vi "p2.vi"() -> ()   [LabVIEW 2023, in "d8.lvlib"]
uses:
  d8.lvlib
  <vilib>/Utility/error.llb/Trim Whitespace One-Sided.vi
  AOC/AOC.lvlib
panel:
  in  "Input":string="LRRLRRRLRRRLLRRLRRLRLRLRRLLRRLRRLRRRLLLRRRLRRRLRRRLLRRRLRRLLRRLRRLRLRRRLRRLRLRRLRRRLLRRLLRLRRRLLRRLRRLLLRLRRRLRLRLRLLRRRLRLLRRRLRLRRRLRRRLLRRLRRRLLRRLRLLRLRRLLLRRLRRLLLRLLRLRRRLRLRLRRRLRRLLRRRLRLRLRRLRRRLRLRRLRRLRRRLRRRLRRRLRRRLRRLLRRLRLLRRLLRRRLRLLRLRLRRLRRLRLRLRRRLRLRLRRLRLRRLRRRR\n\nFPF = (PTN, MPT)\nDGM = (KXM, PRM)\nFKB = (JLC, MBX)\nXCJ = (DCJ, TSH)\nJVH = (VCH, SMV)\nBXL = (HLB, NVF)\nGVD = (FSQ, MFD)\nCDJ = (SMM, HHS)\nBGM = (FHB, LKH)\nFBP = (HHS, SMM)\nLTK = (TCV, GQX)\nLDM = (MRM, JKJ)\nRDK = (KBL, GHP)\nBJB = (XBN, BXG)\nKST = (BGX, VFS)\nVKM = (MFR, CJP)\nCSG = (GGJ, JHH)\nJFS = (QCG, XFR)\nMDV = (FPQ, NRX)\nQHF = (PJP, QHX)\nDHM = (LJC, PDS)\nMMV = (CHS, FXX)\nCQP = (LFN, GSD)\nRDT = (NVG, NVG)\nXFN = (HFM, LTK)\nMFD = (RKJ, XGN)\nDTD = (JBV, JBV)\nKJG = (PCC, PPR)\nGLH = (JRN, BLK)\nKBV = (MCQ, MCS)\nLQF = (KDR, GFC)\nGGB = (JGL, RRM)\nBQX = (QKQ, NSG)\nSVS = (SQL, FXL)\nGMC = (BHG, GPC)\nKPZ = (HLV, RVH)\nRQB = (TDV, XPN)\nGVR = (SXD, QRB)\nMNX = (DLT, CMJ)\nQDM = (TKN, VDH)\nCCB = (KPR, QCK)\nBVF = (QJX, FKK)\nTJB = (HKV, BCP)\nBHC = (SSN, HHH)\nNTN = (RPT, PVF)\nNDP = (BJQ, MGH)\nPJP = (NTN, FSR)\nBLL = (MTQ, SNQ)\nRNP = (RTD, PGM)\nPVF = (BMP, LPM)\nQFL = (NNS, GLR)\nVRG = (GGV, DMG)\nXRX = (TTR, LXS)\nMBH = (RHX, GKF)\nCXD = (LFN, GSD)\nFFK = (LDG, VHS)\nNHM = (BLM, XQD)\nTNB = (KSS, FSB)\nVLX = (KCF, VXL)\nDDF = (TNK, FBS)\nGQR = (BGM, MGR)\nBPQ = (FHD, MJT)\nKPR = (SDL, NMQ)\nCNL = (QFP, XPV)\nHVA = (BRQ, XPL)\nPHF = (LHF, HVR)\nTNZ = (XCM, BFL)\nNDJ = (GCQ, RTL)\nHCT = (PQT, VVB)\nJNH = (GVV, JMC)\nCNV = (SDP, NQR)\nGGV = (RHT, SLG)\nPRX = (FSD, KST)\nBLM = (KKQ, CSG)\nJRN = (GGK, GBF)\nDJK = (GQJ, JKB)\nRVH = (FXJ, JVN)\nRXF = (CHG, GDT)\nMBX = (KJM, XFN)\nHLV = (JVN, FXJ)\nXDG = (HJM, KCT)\nLPM = (RCG, RHG)\nGLP = (XDM, XNC)\nHQP = (JXQ, XPT)\nCXF = (SCV, PHF)\nQJT = (FJN, GHV)\nMPL = (HSQ, FKN)\nSDP = (LCQ, GRV)\nCDQ = (JLV, LLD)\nHHA = (BFL, XCM)\nGPS = (VLX, CPL)\nBXZ = (KSN, VKP)\nPGM = (LJV, CDQ)\nPKG = (VQF, FXC)\nXPL = (LBN, DMV)\nBJJ = (TVV, MNX)\nHLB = (SNN, HNH)\nCDV = (TNB, FSN)\nFXC = (CLF, HSC)\nJFM = (LSR, CNL)\nCMV = (DHQ, DJR)\nLDN = (BCQ, JMS)\nXNC = (JLS, KXS)\nSNN = (NGM, MFJ)\nCND = (RDL, GJJ)\nSKT = (FCM, MRC)\nQRB = (BCG, HRR)\nXNK = (LJC, PDS)\nDGK = (KBF, SRB)\nLNL = (FSD, KST)\nPCM = (PDL, JFS)\nBSV = (LSR, CNL)\nSMX = (TKL, QPF)\nXMS = (MDB, PKP)\nXPT = (LDM, PKV)\nRLB = (XFT, PKM)\nVVV = (NRX, FPQ)\nMGB = (LNN, NKR)\nSFJ = (LFT, QDM)\nMFX = (GLP, RPN)\nDLX = (SQQ, NHM)\nXQC = (HQJ, NPC)\nGHF = (VNG, TGQ)\nLRX = (GDT, CHG)\nSHV = (SRM, DVJ)\nTQS = (PRD, HGV)\nSQK = (QNB, PSJ)\nCHS = (MXK, GCR)\nVDH = (FMX, XMR)\nDGN = (LGT, PNQ)\nRMM = (CFK, RQD)\nRQK = (FSN, TNB)\nSLH = (BDS, BBP)\nHVR = (NTS, NQG)\nPSJ = (JFK, XXM)\nGBD = (VMR, KJG)\nFRH = (MNX, TVV)\nTHH = (GHF, MNF)\nXTP = (VPC, BQQ)\nVMR = (PCC, PPR)\nPPQ = (GJJ, RDL)\nVHK = (TXT, DDN)\nJCG = (CCD, BXL)\nLCQ = (MPF, NDP)\nKCR = (PFH, DJK)\nLHL = (LGL, KCR)\nJMC = (RBG, CGH)\nJPM = (XMS, CVR)\nCLF = (HDT, DHR)\nFSQ = (XGN, RKJ)\nDVJ = (VHD, XNM)\nKCT = (SKT, QLK)\nXFD = (HXR, JVH)\nBVA = (GPT, RSD)\nMGR = (FHB, LKH)\nPXV = (MJJ, VBK)\nFNG = (TQS, HHM)\nGFD = (XRG, JCS)\nSST = (PHP, JGC)\nKJV = (DMG, GGV)\nPQM = (TTX, RMM)\nXRT = (KBL, GHP)\nJLV = (NKV, BLL)\nFKS = (CBR, RLJ)\nHMD = (JNH, GXG)\nFRL = (KQX, DDB)\nTRP = (LXT, HMC)\nTNK = (FRN, FRN)\nKDR = (PRX, LNL)\nXTS = (NDJ, HFB)\nHVM = (FMG, FHN)\nCHH = (TMD, MNM)\nHHM = (PRD, HGV)\nPJC = (FCC, VJD)\nTSH = (RPR, CVJ)\nGGJ = (NFK, NXD)\nDMG = (RHT, SLG)\nQPT = (QFL, PFN)\nDDN = (RHP, NSS)\nXHJ = (BPQ, CSM)\nNNM = (KHG, SRF)\nLFL = (TMN, JCG)\nNKV = (SNQ, MTQ)\nTMH = (LGT, PNQ)\nCCD = (HLB, NVF)\nGSD = (MRB, TFS)\nRHG = (VXH, MXS)\nLFT = (TKN, VDH)\nBJV = (DST, PTK)\nCGD = (PKG, ZZZ)\nVNG = (BJV, HDX)\nHJS = (GPC, BHG)\nFRN = (VKP, KSN)\nMRC = (JKK, CMV)\nBQQ = (NBF, PJC)\nKSN = (FNJ, GVR)\nQNB = (XXM, JFK)\nRSC = (JCB, JCB)\nGCQ = (XGH, FKB)\nSHS = (JBV, DDF)\nLLR = (XHJ, PGB)\nRSA = (RVH, HLV)\nDMX = (GSH, SST)\nHRD = (HLK, DJG)\nLHF = (NTS, NQG)\nJMS = (FKS, HPB)\nSRB = (SRG, GSF)\nLHN = (HLK, DJG)\nDTM = (RXM, VHK)\nPNP = (SNC, LPF)\nMPF = (BJQ, BJQ)\nSCV = (LHF, HVR)\nBTV = (GLH, PNN)\nNJG = (RXK, NXB)\nNGM = (THG, TXQ)\nFXL = (XRX, MBV)\nNHJ = (DSX, NNM)\nRBG = (DGK, LFQ)\nHGV = (HTS, RNP)\nLDF = (KRB, NXC)\nPMR = (GNH, CHQ)\nDVM = (MNM, TMD)\nFBS = (FRN, BXZ)\nBMM = (XSK, DDK)\nGGK = (MXH, JNG)\nNXB = (LHN, HRD)\nPNN = (JRN, BLK)\nPSV = (LLR, KXX)\nKGK = (TJP, QMM)\nCVG = (VLX, CPL)\nQNF = (XPB, PCM)\nHTS = (PGM, RTD)\nFJN = (DTD, SHS)\nJXB = (CLX, KPZ)\nDLT = (JGH, SFD)\nSFV = (HJM, KCT)\nGSF = (DLX, CHL)\nTKN = (XMR, FMX)\nLJB = (QJT, FVJ)\nQFP = (NXL, DGP)\nPKV = (JKJ, MRM)\nRHX = (RDK, XRT)\nKDP = (FKN, HSQ)\nRLJ = (BGF, JRP)\nVQR = (FDK, RLB)\nXNX = (HGQ, HGQ)\nDSX = (KHG, SRF)\nPDS = (VQK, KNJ)\nGKX = (TKL, QPF)\nCHQ = (XSM, HMD)\nKXX = (XHJ, PGB)\nMDB = (VVV, MDV)\nBCG = (XJX, SQK)\nKJM = (LTK, HFM)\nHRR = (SQK, XJX)\nGXD = (JFM, BSV)\nSCR = (JDN, QRS)\nGMK = (FPF, CTM)\nKXM = (PDJ, MFX)\nDKQ = (GCL, QFN)\nDJR = (FGV, PSV)\nGQX = (DFL, LQF)\nPTK = (TRS, TMC)\nBLK = (GGK, GBF)\nRSD = (XDG, SFV)\nSVT = (PXV, XCL)\nXFT = (BJJ, FRH)\nLSR = (XPV, QFP)\nBCP = (NMB, NXM)\nKGP = (RDT, FNB)\nDHF = (PNN, GLH)\nJHH = (NXD, NFK)\nDGP = (GKX, SMX)\nKSK = (DKP, RXT)\nKRM = (PQM, DCK)\nXJX = (QNB, PSJ)\nJKK = (DJR, DHQ)\nCFK = (DGN, TMH)\nPSS = (HNP, STL)\nMFR = (PMR, RJS)\nJNG = (TQQ, HXB)\nMDG = (VCC, HTF)\nVCC = (DGM, MKH)\nTQQ = (FCQ, SCR)\nDMK = (GXD, GFF)\nGHV = (DTD, SHS)\nHLP = (NNH, TQN)\nBGK = (QHJ, BQX)\nVKN = (DPT, FNG)\nSTL = (DPP, NMX)\nQFS = (MGR, BGM)\nHSC = (DHR, HDT)\nFPQ = (NSL, RQN)\nQMM = (CDJ, FBP)\nPDL = (XFR, QCG)\nPDJ = (GLP, RPN)\nFSD = (VFS, BGX)\nMPT = (DKQ, RSQ)\nMHQ = (NTL, TKG)\nMPC = (NQJ, NQJ)\nDST = (TRS, TMC)\nKHD = (CLX, CLX)\nBNT = (MFR, CJP)\nVJD = (GPS, CVG)\nDLG = (JCS, XRG)\nMCD = (CHH, DVM)\nVSG = (XPR, TVQ)\nMSX = (VQR, KXQ)\nVMV = (VQR, KXQ)\nQCG = (NHJ, NMH)\nRPN = (XNC, XDM)\nNVG = (RSC, RSC)\nGDT = (LDC, QPT)\nGMX = (RJX, VRM)\nRDL = (MBH, NTF)\nXXM = (JSC, MHQ)\nSRF = (BGK, NQF)\nXNM = (SGJ, XCJ)\nRPT = (LPM, BMP)\nGPT = (SFV, XDG)\nJCB = (BFL, XCM)\nQKQ = (FRL, GGT)\nMTQ = (LQB, XPG)\nCHG = (QPT, LDC)\nFMS = (FJX, GMX)\nMBV = (LXS, TTR)\nJFP = (XPN, TDV)\nJFJ = (HNP, STL)\nGKF = (RDK, XRT)\nLDK = (QCT, TVX)\nCLX = (RVH, HLV)\nTXQ = (DFR, KQF)\nXGH = (MBX, JLC)\nKFB = (SHV, MRV)\nRSV = (GSX, TPK)\nNKR = (KFB, TFN)\nFCQ = (JDN, QRS)\nRQN = (TLC, GFQ)\nFSN = (FSB, KSS)\nQDQ = (VBQ, GSM)\nFFC = (DKC, DMK)\nKBC = (BHQ, TRP)\nPHB = (VCC, HTF)\nGBH = (FFC, CGL)\nTTR = (KBV, LJP)\nMRB = (DHG, QNF)\nSDL = (PSS, JFJ)\nTMC = (BXK, RSV)\nLXT = (GGB, MDT)\nLQB = (BNT, VKM)\nRXT = (GBH, SSD)\nSSN = (CRH, XTP)\nMRV = (SRM, DVJ)\nFJX = (RJX, VRM)\nFQB = (MNF, GHF)\nDKC = (GFF, GXD)\nMGQ = (LDK, RVG)\nDLK = (FPF, CTM)\nFHN = (HKK, BVF)\nBFL = (LJG, XQM)\nPKP = (VVV, MDV)\nQHJ = (QKQ, NSG)\nBCQ = (HPB, FKS)\nLDG = (VMV, MSX)\nBFH = (RXT, DKP)\nXPB = (JFS, PDL)\nHDX = (PTK, DST)\nNQF = (BQX, QHJ)\nDPT = (TQS, HHM)\nDCK = (TTX, RMM)\nNPC = (KGP, QJG)\nBCD = (NXB, RXK)\nHDT = (HPM, FTQ)\nFHD = (XNK, DHM)\nNNS = (XFD, MBT)\nGSX = (VRG, KJV)\nBXG = (BFH, KSK)\nVVB = (QDQ, JXC)\nNVF = (HNH, SNN)\nKRB = (JBH, JNJ)\nFXX = (GCR, MXK)\nJXQ = (LDM, PKV)\nMTT = (DLG, GFD)\nHXR = (VCH, SMV)\nMNM = (SPQ, PNP)\nQJG = (RDT, FNB)\nJLS = (KRM, LBQ)\nCJK = (TJB, VDD)\nTXT = (RHP, NSS)\nFXT = (JMS, BCQ)\nNSS = (LRX, RXF)\nVJQ = (RSC, MXR)\nXXH = (LNN, NKR)\nNSL = (GFQ, TLC)\nXSM = (GXG, JNH)\nHFM = (TCV, GQX)\nJGC = (NDL, JPM)\nHGQ = (GPT, RSD)\nCHL = (SQQ, NHM)\nVBK = (GKG, XTS)\nMBT = (HXR, JVH)\nFNJ = (SXD, QRB)\nJBH = (HCT, SGG)\nJRP = (FXP, VKN)\nVRM = (MPC, GQP)\nBBP = (JCL, LDF)\nGXH = (RXM, VHK)\nMXR = (JCB, TNZ)\nBSD = (CCP, GBD)\nQFN = (MPL, KDP)\nLNN = (TFN, KFB)\nSQQ = (BLM, XQD)\nMJT = (XNK, DHM)\nGSH = (JGC, PHP)\nPQT = (JXC, QDQ)\nRVG = (QCT, TVX)\nDHG = (PCM, XPB)\nLKJ = (HQP, HHG)\nXHB = (SJL, DMX)\nGKG = (HFB, NDJ)\nPGB = (BPQ, CSM)\nVBQ = (CVS, QHF)\nJXC = (GSM, VBQ)\nQCK = (SDL, NMQ)\nPFN = (NNS, GLR)\nRXK = (LHN, HRD)\nBVX = (GMK, DLK)\nLPF = (MMV, LQK)\nSMM = (SFJ, KGR)\nSJL = (SST, GSH)\nHMC = (MDT, GGB)\nVQF = (CLF, HSC)\nNRX = (RQN, NSL)\nCBR = (JRP, BGF)\nJLC = (KJM, XFN)\nTMD = (SPQ, PNP)\nHXB = (FCQ, SCR)\nSBQ = (SQV, NCH)\nLGT = (MGB, XXH)\nHSF = (TJB, VDD)\nJBS = (MGQ, NVQ)\nDKP = (SSD, GBH)\nHSQ = (SVT, LKV)\nGPC = (HVM, TGC)\nTVV = (DLT, CMJ)\nBHG = (TGC, HVM)\nCGR = (LDN, FXT)\nPFH = (GQJ, GQJ)\nFCM = (JKK, CMV)\nRRM = (KJP, BMM)\nFCG = (MDG, PHB)\nMCS = (HLP, DNV)\nBXK = (GSX, TPK)\nVQK = (HJS, GMC)\nLDH = (XPR, TVQ)\nDXN = (GMK, DLK)\nGFQ = (RQB, JFP)\nPKK = (BBP, BDS)\nBBR = (FXT, LDN)\nBJQ = (KHD, KHD)\nRCG = (MXS, VXH)\nHPM = (KJF, CXF)\nQJX = (CDV, RQK)\nNMB = (RKC, GVD)\nJCL = (KRB, NXC)\nGXM = (BBR, CGR)\nNMX = (XNX, SQP)\nNXM = (RKC, GVD)\nQMT = (MDG, PHB)\nDMV = (LTG, SBQ)\nFTQ = (KJF, CXF)\nTCV = (DFL, LQF)\nMFJ = (TXQ, THG)\nVKP = (FNJ, GVR)\nXQD = (CSG, KKQ)\nSRM = (VHD, XNM)\nSLG = (LRJ, JFL)\nJCS = (CQP, CXD)\nLJP = (MCQ, MCS)\nNBF = (FCC, VJD)\nDFL = (KDR, GFC)\nNFM = (XBN, BXG)\nCMR = (PKG, PKG)\nJVN = (XHB, MCC)\nRKC = (FSQ, MFD)\nJKJ = (BSQ, LJB)\nBGX = (MMD, FMS)\nTHG = (KQF, DFR)\nRKJ = (CVN, FFK)\nLQK = (CHS, FXX)\nCPL = (VXL, KCF)\nJSC = (TKG, NTL)\nDNV = (TQN, NNH)\nLFF = (HQJ, NPC)\nTVQ = (SSF, GXM)\nNQR = (LCQ, GRV)\nTMN = (BXL, CCD)\nXDM = (KXS, JLS)\nCJP = (RJS, PMR)\nHKV = (NMB, NXM)\nSPQ = (SNC, LPF)\nHQJ = (KGP, QJG)\nGXG = (JMC, GVV)\nKSS = (CND, PPQ)\nLJG = (DTM, GXH)\nBHQ = (HMC, LXT)\nFGV = (KXX, LLR)\nKCF = (LKJ, NTJ)\nPRM = (MFX, PDJ)\nQKD = (FXL, SQL)\nDDB = (CSB, MCD)\nVHH = (CMR, CGD)\nLLM = (BVX, DXN)\nPTN = (RSQ, DKQ)\nGSM = (CVS, QHF)\nCVN = (VHS, LDG)\nRHT = (LRJ, JFL)\nJFK = (JSC, MHQ)\nNTS = (QFS, GQR)\nTQN = (DHF, BTV)\nKHG = (BGK, NQF)\nZZZ = (FXC, VQF)\nVXL = (NTJ, LKJ)\nVFS = (MMD, FMS)\nLBQ = (PQM, DCK)\nKQX = (CSB, MCD)\nFDK = (XFT, PKM)\nNQG = (GQR, QFS)\nKXS = (LBQ, KRM)\nJDN = (HDL, CCB)\nTKL = (HSF, CJK)\nXRG = (CQP, CXD)\nBMP = (RCG, RHG)\nKQF = (KGK, LGN)\nHLK = (MTT, PFT)\nNFK = (MRS, CNV)\nHNH = (MFJ, NGM)\nFKN = (SVT, LKV)\nVPC = (PJC, NBF)\nDDK = (SVS, QKD)\nDCJ = (RPR, CVJ)\nNQJ = (CMR, CMR)\nLGL = (PFH, PFH)\nRTD = (CDQ, LJV)\nFVJ = (FJN, GHV)\nBDS = (LDF, JCL)\nNSG = (GGT, FRL)\nRXM = (DDN, TXT)\nJNJ = (SGG, HCT)\nSRG = (DLX, CHL)\nTGC = (FMG, FHN)\nFMG = (BVF, HKK)\nNTJ = (HHG, HQP)\nKNJ = (HJS, GMC)\nQJB = (CCP, GBD)\nNXL = (SMX, GKX)\nVHS = (MSX, VMV)\nCRH = (BQQ, VPC)\nGFF = (JFM, BSV)\nGLR = (XFD, MBT)\nXPR = (GXM, SSF)\nLLD = (BLL, NKV)\nKXQ = (FDK, RLB)\nMXH = (TQQ, HXB)\nRQD = (DGN, TMH)\nFNB = (NVG, VJQ)\nMGH = (KHD, JXB)\nJGL = (BMM, KJP)\nKJF = (SCV, PHF)\nSXD = (BCG, HRR)\nTPK = (KJV, VRG)\nTJP = (FBP, CDJ)\nMKH = (KXM, PRM)\nHJM = (SKT, QLK)\nGHP = (RFL, KBC)\nLGN = (TJP, QMM)\nLJV = (JLV, LLD)\nNXD = (CNV, MRS)\nLKH = (LLM, BNK)\nCTM = (MPT, PTN)\nSNC = (LQK, MMV)\nPNQ = (XXH, MGB)\nFMX = (BSD, QJB)\nQQL = (HHH, SSN)\nQLK = (FCM, MRC)\nCMJ = (JGH, SFD)\nFHB = (BNK, LLM)\nTKG = (FQB, THH)\nXPV = (DGP, NXL)\nRHP = (LRX, RXF)\nBRQ = (LBN, DMV)\nNDL = (XMS, CVR)\nLDC = (PFN, QFL)\nDPP = (XNX, XNX)\nNMQ = (PSS, JFJ)\nSGG = (PQT, VVB)\nFSR = (RPT, PVF)\nAAA = (VQF, FXC)\nJFL = (BJB, NFM)\nXFR = (NHJ, NMH)\nHHS = (SFJ, KGR)\nMLZ = (RSD, GPT)\nMNF = (VNG, TGQ)\nFXP = (DPT, FNG)\nMRS = (SDP, NQR)\nMDT = (JGL, RRM)\nMJJ = (GKG, XTS)\nPFT = (GFD, DLG)\nTVX = (BCD, NJG)\nNPA = (VKP, KSN)\nTDV = (LDH, VSG)\nGQJ = (PDM, PDM)\nNTF = (GKF, RHX)\nGGT = (KQX, DDB)\nLFN = (TFS, MRB)\nCSM = (MJT, FHD)\nNVQ = (RVG, LDK)\nPKM = (FRH, BJJ)\nPDM = (BRQ, XPL)\nJGH = (BHC, QQL)\nSSF = (CGR, BBR)\nGVV = (CGH, RBG)\nFSB = (PPQ, CND)\nLKV = (XCL, PXV)\nMXK = (SLH, PKK)\nSQL = (XRX, MBV)\nLRJ = (BJB, NFM)\nVXH = (LFF, XQC)\nHTF = (MKH, DGM)\nCTB = (LGL, KCR)\nHFB = (RTL, GCQ)\nNTL = (FQB, THH)\nSFD = (QQL, BHC)\nHNP = (DPP, DPP)\nTTX = (RQD, CFK)\nMCQ = (HLP, DNV)\nCCP = (VMR, KJG)\nTFN = (MRV, SHV)\nJKB = (PDM, RFZ)\nTGQ = (BJV, HDX)\nPHP = (JPM, NDL)\nRJX = (MPC, GQP)\nCVJ = (LFL, KLG)\nKJP = (DDK, XSK)\nQPF = (HSF, CJK)\nSNQ = (XPG, LQB)\nBGF = (VKN, FXP)\nKLG = (TMN, JCG)\nCGL = (DMK, DKC)\nXCM = (XQM, LJG)\nRPR = (LFL, KLG)\nLFQ = (KBF, SRB)\nRJS = (CHQ, GNH)\nHDL = (KPR, QCK)\nFXJ = (MCC, XHB)\nXPG = (VKM, BNT)\nDHQ = (FGV, PSV)\nSQV = (QMT, FCG)\nDHR = (FTQ, HPM)\nFCC = (GPS, CVG)\nNCH = (FCG, QMT)\nQRS = (HDL, CCB)\nXQM = (GXH, DTM)\nSGJ = (TSH, DCJ)\nKBL = (RFL, KBC)\nNXC = (JBH, JNJ)\nBSQ = (QJT, FVJ)\nLTG = (NCH, SQV)\nSMV = (JBS, MDQ)\nGJJ = (MBH, NTF)\nGRV = (MPF, NDP)\nHPB = (RLJ, CBR)\nTRS = (BXK, RSV)\nGCR = (SLH, PKK)\nHHH = (CRH, XTP)\nGNH = (XSM, HMD)\nRSQ = (QFN, GCL)\nHKK = (QJX, FKK)\nJBV = (TNK, TNK)\nTFS = (DHG, QNF)\nRTL = (FKB, XGH)\nHHG = (XPT, JXQ)\nPPR = (LHL, CTB)\nSQP = (HGQ, MLZ)\nXBN = (BFH, KSK)\nCVR = (MDB, PKP)\nRFL = (BHQ, TRP)\nQHX = (FSR, NTN)\nVCH = (MDQ, JBS)\nGCL = (MPL, KDP)\nKKQ = (GGJ, JHH)\nGFC = (PRX, LNL)\nPRD = (HTS, RNP)\nGQP = (NQJ, VHH)\nLJC = (VQK, KNJ)\nQCT = (BCD, NJG)\nKBF = (SRG, GSF)\nNNH = (BTV, DHF)\nSSD = (CGL, FFC)\nVDD = (HKV, BCP)\nVHD = (XCJ, SGJ)\nRFZ = (XPL, BRQ)\nKGR = (LFT, QDM)\nMDQ = (NVQ, MGQ)\nMXS = (LFF, XQC)\nPCC = (LHL, CTB)\nTLC = (RQB, JFP)\nCVS = (PJP, QHX)\nBNK = (DXN, BVX)\nCSB = (CHH, DVM)\nXPN = (VSG, LDH)\nXSK = (SVS, QKD)\nLBN = (LTG, SBQ)\nFKK = (RQK, CDV)\nMCC = (SJL, DMX)\nNMH = (DSX, NNM)\nMMD = (GMX, FJX)\nLXS = (LJP, KBV)\nXMR = (QJB, BSD)\nDFR = (KGK, LGN)\nDJG = (PFT, MTT)\nCGH = (DGK, LFQ)\nMRM = (BSQ, LJB)\nXCL = (MJJ, VBK)\nGBF = (JNG, MXH)\nXGN = (FFK, CVN)"
  in  "Example":string="LR\n\n11A = (11B, XXX)\n11B = (XXX, 11Z)\n11Z = (11B, XXX)\n22A = (22B, XXX)\n22B = (22C, 22C)\n22C = (22Z, 22Z)\n22Z = (22B, 22B)\nXXX = (XXX, XXX)"
  in  "Example":bool
  out "Answer":u64=12030780859469
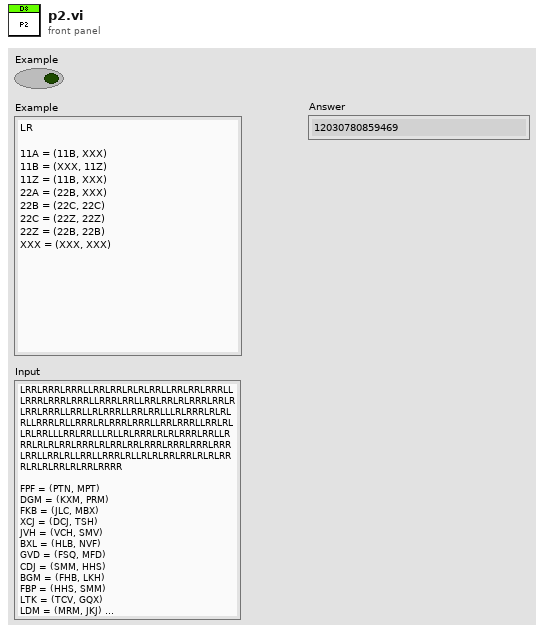
[diagram p1: front panel]
types:
  T1 = cluster{string, "index of element":i32, "index of element":i32}
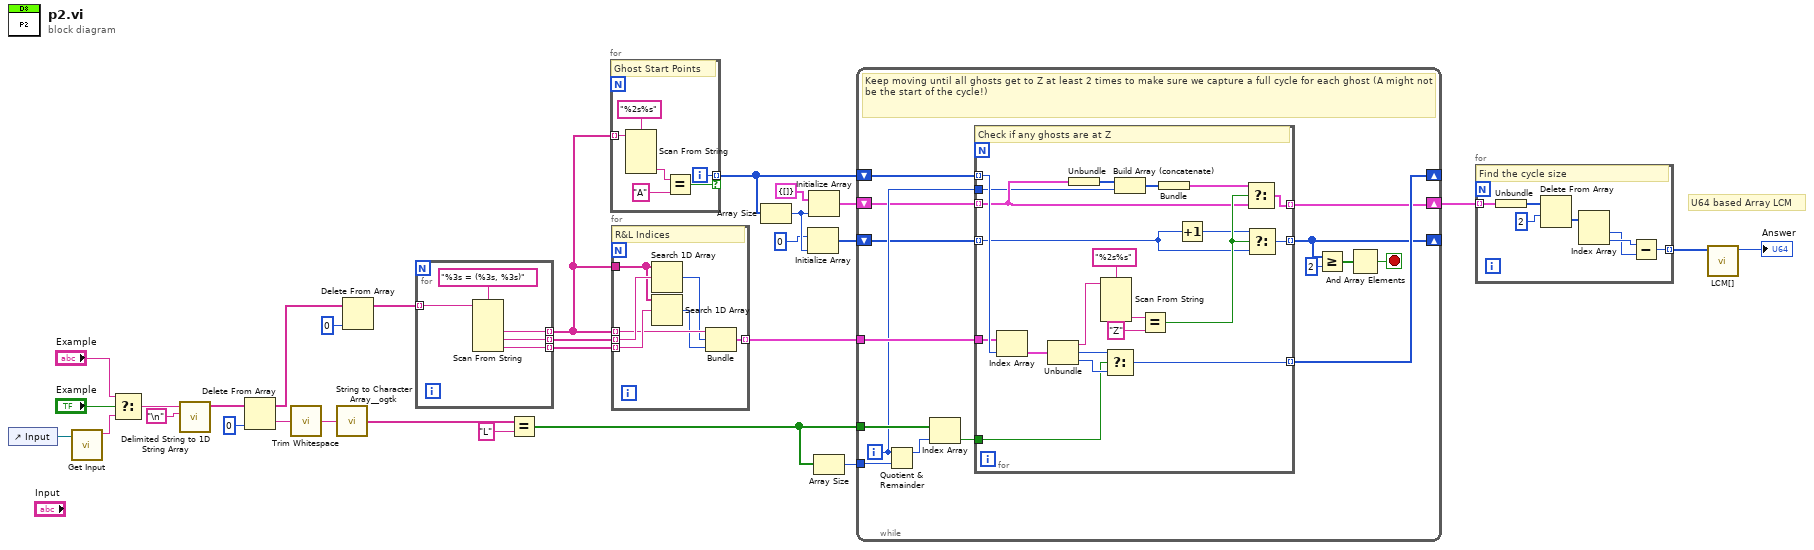
[diagram p0: block diagram]
diagram:
  # "U64 based Array LCM"
  n1 = control-ref of="Input"() -> (w26:refnum<vi>)
  n2 = call "Get Input.vi"("Input ref"=w26) -> ("Input"=w30:string)  [unwired: 10 in]
  n3 = Select(t="Example", s="Example", f=w30) -> (s? t:f=w29:string)
  n4 = call <vilib>:"Delimited String to 1D String Array.vi"("delimiter"="\n", "delimited string"=w29) -> ("string array"=w25:string[])  [unwired: 9 in]
  n5 = Delete From Array(array=w25, index=0) -> (deleted portion=w22:string, array with subset deleted=w23:string[])  [unwired: 1 in]
  n6 = call <vilib>:"Trim Whitespace.vi"("string"=w22) -> ("trimmed string"=w21:string)  [unwired: 1 in]
  n7 = call <userlib>:"String to Character Array__ogtk.vi"("Input String"=w21) -> ("Character Array"=w16:string[])
  n8 = Delete From Array(array=w23, index=0) -> (array with subset deleted=w20:string[])  [unwired: 1 in, 1 out]
  n9 = for {
    tunnel: w20 -> [w35] mode=indexing
    tunnel: [w33] -> w11 mode=indexing
    tunnel: [w32] -> w19 mode=indexing
    tunnel: [w31] -> w18 mode=indexing
    n10 = Scan From String(format string="%3s = (%3s, %3s)", input string=w35) -> (output 1=w33:string, output 2=w32:string, output 3=w31:string)  [unwired: 5 in, 3 out]
  }
  n11 = Equal?(x=w16, y="L") -> (x = y?=w15:bool[])
  n12 = for {
    tunnel: w11 -> [w40] mode=indexing
    tunnel: [w41] -> w10 mode=indexing if=w36
    i -> [w41]
    # "Ghost Start Points"
    n13 = Scan From String(format string="%2s%s", input string=w40) -> (output 2=w38:string)  [unwired: 5 in, 3 out]
    n14 = Equal?(x=w38, y="A" ("element")) -> (x = y?=w36:bool)
  }
  n15 = for {
    tunnel: w11 -> [w47]
    tunnel: w19 -> [w48] mode=indexing
    tunnel: w18 -> [w46] mode=indexing
    tunnel: w11 -> [w45] mode=indexing
    tunnel: [w42] -> w17 mode=indexing
    # "R&L Indices"
    n16 = Search 1D Array(1D array=w47, element=w48) -> (index of element=w44:i32)  [unwired: 1 in]
    n17 = Search 1D Array(1D array=w47, element=w46) -> (index of element=w43:i32)  [unwired: 1 in]
    n18 = Bundle(w45, "index of element"=w44, "index of element"=w43) -> (w42:T1)  [unwired: 1 in]
  }
  n19 = Array Size(array=w10) -> (size(s)=w8:i32)
  n20 = Initialize Array(u64 0, w8) -> (w7:u64[])
  n21 = Initialize Array(cluster{u64[]} {[]}, w8) -> (w9:cluster{u64[]}[])
  n22 = Array Size(array=w15) -> (size(s)=w24:i32)
  n23 = while {
    tunnel: w15 -> [w63]
    tunnel: w24 -> [w62]
    tunnel: w17 -> [w59]
    shift-right: [w58] -> _
    shift-left: w10 -> [w60]
    shift-right: [w51] -> _
    shift-left: w7 -> [w54]
    shift-right: [w53] -> w4
    shift-left: w9 -> [w55]
    i -> [w56]
    stop <- w49 stop-if-true
    # "Keep moving until all ghosts get to Z at least 2 times to make sure we capture a full cycle for each ghost (A might not be the start of the cycle!)"
    n24 = Quotient & Remainder(x=w56, y=w62) -> (x-y*floor(x/y)=w61:i32)  [unwired: 1 out]
    n25 = Index Array(array=w63, index=w61) -> (element=w57:bool)
    n26 = for {
      tunnel: w60 -> [w78] mode=indexing
      tunnel: w59 -> [w77]
      tunnel: [w75] -> w58 mode=indexing
      tunnel: w57 -> [w74]
      tunnel: w56 -> [w65]
      tunnel: w55 -> [w68] mode=indexing
      tunnel: w54 -> [w70] mode=indexing
      tunnel: [w72] -> w51 mode=indexing
      tunnel: [w73] -> w53 mode=indexing
      # "Check if any ghosts are at Z"
      n27 = Index Array(array=w77, index=w78) -> (element=w81:T1)
      n28 = Unbundle(w81) -> (w76:string, "index of element"=w80:i32, "index of element"=w79:i32)
      n29 = Unbundle(w68) -> (w67:u64[])
      n30 = Scan From String(format string="%2s%s", input string=w76) -> (output 2=w83:string)  [unwired: 5 in, 3 out]
      n31 = Select(t=w80, s=w74, f=w79) -> (s? t:f=w75:i32)
      n32 = Build Array (concatenate)(w67, w65) -> (w66:u64[])
      n33 = Equal?(x=w83, y="Z" ("element")) -> (x = y?=w71:bool)
      n34 = Bundle(w66) -> (w64:cluster{u64[]})  [unwired: 1 in]
      n35 = Increment(x=w70) -> (x+1=w69:u64)
      n36 = Select(t=w64, s=w71, f=w68) -> (s? t:f=w73:cluster{u64[]})
      n37 = Select(t=w69, s=w71, f=w70) -> (s? t:f=w72:u64)
    }
    n38 = Greater Or Equal?(x=w51, y=u64 2) -> (x >= y?=w52:bool[])
    n39 = And Array Elements(Boolean array=w52) -> (logical AND=w49:bool)
  }
  n40 = for {
    tunnel: w4 -> [w91] mode=indexing
    tunnel: [w85] -> w2 mode=indexing
    # "Find the cycle size"
    n41 = Unbundle(w91) -> (w90:u64[])
    n42 = Delete From Array(array=w90, length=2) -> (deleted portion=w88:u64[])  [unwired: 1 in, 1 out]
    n43 = Index Array(array=w88) -> (element #1=w86:u64, element #2=w87:u64)  [unwired: 2 in]
    n44 = Subtract(x=w87, y=w86) -> (x-y=w85:u64)
  }
  n45 = call "LCM[].vi"("Array"=w2) -> ("LCM"=→"Answer":u64)  [unwired: 10 in]
